vi "Invisible Processes.vi"(8 "error in":errorcluster, 10 "Server Name":string="localhost", 11 "Current Hiden Processes":string[](array[string])) -> (0 "error out":errorcluster, 3 "Invis Libraries":string[](array[string]))   [LabVIEW 2014]
doc: "<B>Copyrights</B>: (c) MHWirth 2015. All rights reserved.\n\nThis subVI allows the user to select those deploed processes that should be hidden."
panel:
  in  "Remove Button":bool
  in  "Add Button":bool
  in  "To Hide":i32(listbox) caption="To hide"
  in  "Deployed Libraries":i32(listbox)
  in  "update":bool
  # "Manage Visible Processes"
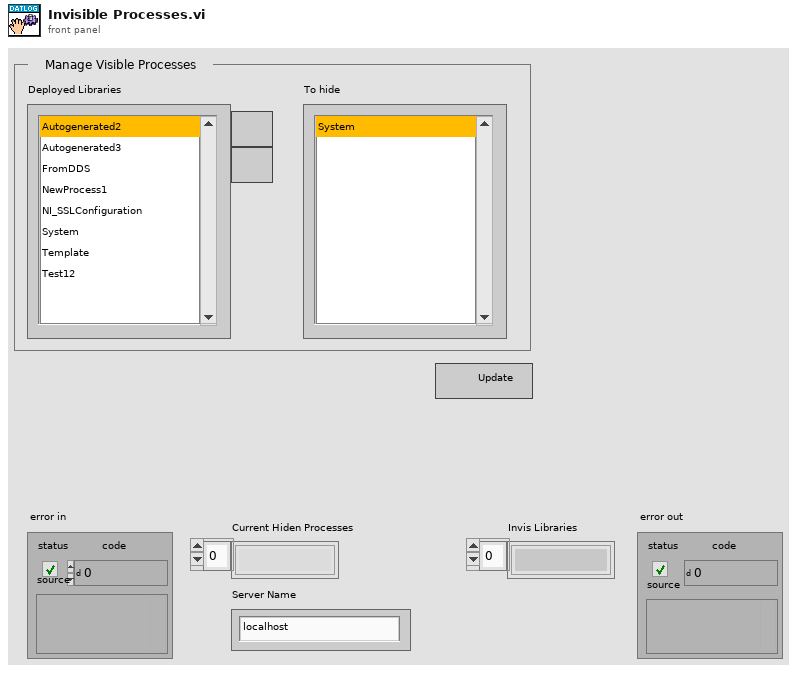
[diagram p1: front panel]
types:
  T1 = cluster{"Library Name":string[], "library URL":string[]}
  T2 = typedef "eventvkey.ctl" = enum16{"ASCII", "Enter", "Return", "Shift", "Ctrl", "Alt", "Cmd", "Opt", "Caps", "NumLock", "Clear", "Break", "Up", "Down", "Left", "Right", "Insert", "Delete", "Home", "End", "PageUp", "PageDown", "Escape", "Help", "Pause", "ScrollLock", "F1", "F2", "F3", "F4", "F5", "F6", "F7", "F8", "F9", "F10", "F11", "F12", "F13", "F14", "F15", "F16", "F17", "F18", "F19", "F20", "F21", "F22", "F23", "F24", "Play", "VolumeUp", "VolumeDown", "Mute", "Two Byte Char"}
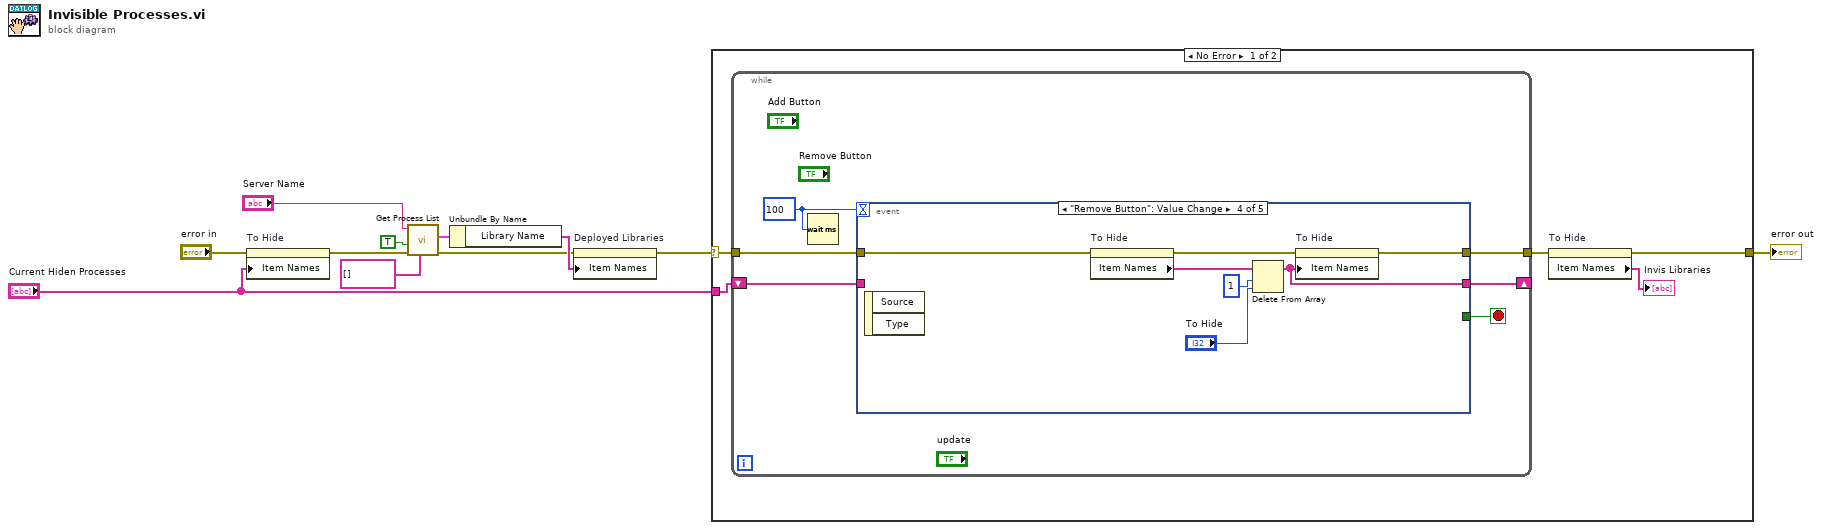
[diagram p0: block diagram]
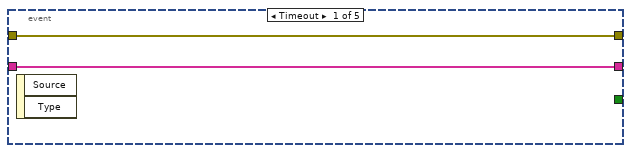
[diagram p2: hidden frame]
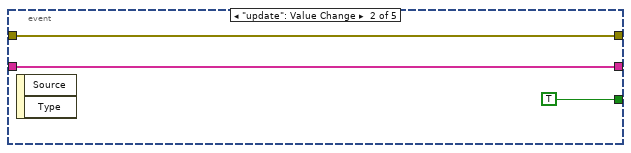
[diagram p3: hidden frame]
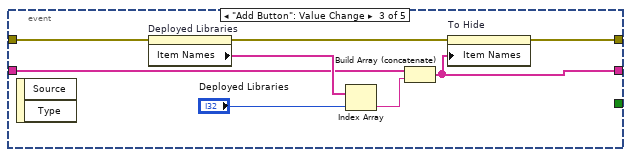
[diagram p4: hidden frame]
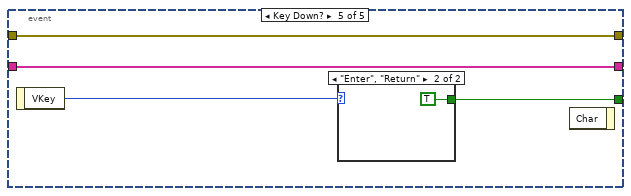
[diagram p5: hidden frame]
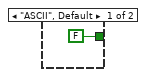
[diagram p6: hidden frame]
diagram:
  n1 = property on="To Hide" class="LstBox (strict)"(error in="error in", "Item Names"="Current Hiden Processes") -> (error out=w1:errorcluster)  [unwired: 1 in, 1 out]
  n2 = call "Get Process List.vi"("Invisible Libraries"=string[] [], "Error In"=w1, "Remove Library"=TRUE ("Remove \"System\" library"), "Server Name"="Server Name") -> ("Error Out"=w6:errorcluster, "Libraries"=w8:T1)  [unwired: 5 in, 1 out]
  n3 = Unbundle By Name(w8) -> ("Library Name"=w7:string[])
  n4 = property on="Deployed Libraries" class="LstBox (strict)"(error in=w6, "Item Names"=w7) -> (error out=w2:errorcluster)  [unwired: 1 in, 1 out]
  n5 = case shown="No Error" w2 {
    selector: w2 -> [w16 w49]
    tunnel: [w14 w49] -> w11
    tunnel: "Current Hiden Processes" -> [w12 _]
    frame No Error {
      n6 = while {
        tunnel: w16 -> [w20]
        tunnel: [w19] -> w15
        shift-right: [w17] -> _
        shift-left: w12 -> [w18]
        stop <- w21 stop-if-true
        w22 = u32 100 ("milliseconds to wait")
        n7 = Wait (ms)(milliseconds to wait=w22) -> ()  [unwired: 1 out]
        n8 = event shown="[3] \"Remove Button\": Value Change" {
          selector: _ -> [_ _ _ _ _]
          dyn-events: _ -> [_ _ _ _ _]
          timeout: w22 -> [_ _ _ _ _]
          tunnel: [_ TRUE _ _ w45] -> w21
          tunnel: w20 -> [w23 w26 w35 w42 w46]
          tunnel: [w23 w26 w30 w41 w46] -> w19
          tunnel: w18 -> [w24 w25 w32 _ w43]
          tunnel: [w24 w25 w28 w36 w43] -> w17
          event Timeout {
            n9 = event-data() -> ()  [unwired: 1 in, 2 out]
          }
          event "update": Value Change {
            n10 = event-data() -> ()  [unwired: 1 in, 2 out]
          }
          event "Add Button": Value Change {
            n11 = event-data() -> ()  [unwired: 1 in, 2 out]
            n12 = property on="Deployed Libraries" class="LstBox (strict)"(error in=w35) -> (error out=w29:errorcluster, "Item Names"=w34:string[])  [unwired: 1 in, 1 out]
            n13 = Index Array(array=w34, index="Deployed Libraries") -> (element=w31:string)
            n14 = Build Array (concatenate)(w32, w31) -> (w28:string[])
            n15 = property on="To Hide" class="LstBox (strict)"(error in=w29, "Item Names"=w28) -> (error out=w30:errorcluster)  [unwired: 1 in, 1 out]
          }
          event "Remove Button": Value Change {
            n16 = event-data() -> ()  [unwired: 1 in, 2 out]
            n17 = property on="To Hide" class="LstBox (strict)"(error in=w42) -> (error out=w40:errorcluster, "Item Names"=w39:string[])  [unwired: 1 in, 1 out]
            n18 = Delete From Array(array=w39, length=1, index="To Hide") -> (array with subset deleted=w36:string[])  [unwired: 1 out]
            n19 = property on="To Hide" class="LstBox (strict)"(error in=w40, "Item Names"=w36) -> (error out=w41:errorcluster)  [unwired: 1 in, 1 out]
          }
          event Key Down? {
            n20 = event-data() -> ("VKey"=w44:T2)  [unwired: 1 in]
            n21 = case shown="\"Enter\", \"Return\"" w44 {
              tunnel: [FALSE TRUE] -> w45
              frame "ASCII", Default {
              }
              frame "Enter", "Return" {
              }
            }
            n22 = event-data() -> ()  [unwired: 2 in, 1 out]
          }
        }
      }
      n23 = property on="To Hide" class="LstBox (strict)"(error in=w15) -> (error out=w14:errorcluster, "Item Names"=→"Invis Libraries":string[])  [unwired: 1 in, 1 out]
    }
    frame Error {
    }
  }
  "error out" <- w11
